vi "Vision Research Phantom Series PhCon PhSetCameraName.vi"(0 "CN in":u32=1, 2 "pCameraName":string, 5 "Error In (no error)":errorcluster) -> (14 "CN out":u32=1, 19 "Error Out":errorcluster)   [LabVIEW 2013, in "VRI.lvlib"]
doc: "PhCon.dll\n\nPhSetCameraName\nHRESULT PhSetCameraName(UINT CN, char *pCameraName);\n\nParameters Description\nCN (in) Camera number.\npCameraName (in) Camera name, maximum 15 char.\nReturn HRESULT (0=Ok)\nComments Let the user change the name of the camera.\n\nWritten by:\nBLOOMY CONTROLS, INC\nWINDSOR, CT 06095, USA\n860-298-9925\nwww.bloomy.com\nV1.0.0\nMay, 2004"
uses:
  VRI.lvlib
  Phantom DLLs/PhCon.dll
panel:
  # "For instructions on the use of this VI, press Ctrl+H to display the help window and move the mouse over the icon, controls, and indicators"
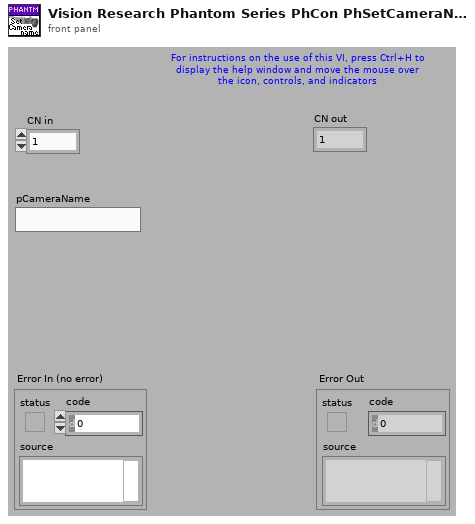
[diagram p1: front panel]
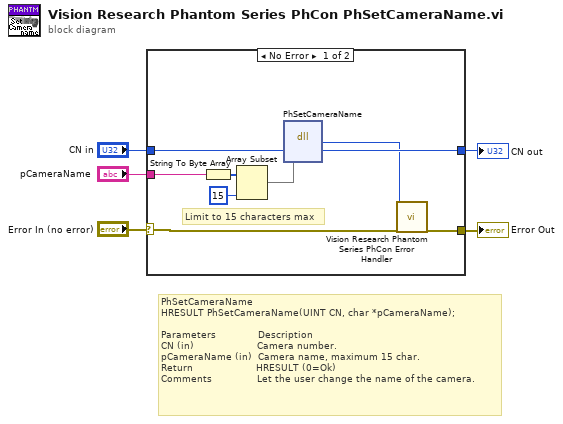
[diagram p0: block diagram]
diagram:
  # "PhSetCameraName\nHRESULT PhSetCameraName(UINT CN, char *pCameraName);\n\nParameters              Description\nCN (in)                     Camera number.\npCameraName (in)  Camera name, maximum 15 char.\nReturn                     HRESULT (0=Ok)\nComments               Let the user change the name of the camera."
  n1 = case shown="No Error" "Error In (no error)" {
    selector: "Error In (no error)" -> [w14 w16]
    tunnel: [w13 w16] -> w4
    tunnel: "CN in" -> [w12 w15]
    tunnel: "pCameraName" -> [w11 _]
    tunnel: [w10 w15] -> w1
    frame No Error {
      # "Limit to 15 characters max"
      n2 = String To Byte Array(string=w11) -> (unsigned byte array=w6:u8[])
      n3 = Array Subset(array=w6, length=15) -> (w8:u8[])  [unwired: 1 in]
      n4 = dll-call lib="C:/Projects/SDK/32-bit/Vision Research Phantom Series Labview Driver/Phantom DLLs/PhCon.dll" fn="PhSetCameraName"("CN"=w12, "pCameraName"=w8) -> ("HRESULT"=w9:i32, "CN"=w10:u32)  [unwired: 3 in, 3 out]
      n5 = call "Vision Research Phantom Series PhCon Error Handler.vi"("ErrNo"=w9, "Error In (no error)"=w14) -> ("Error Out"=w13:errorcluster)  [unwired: 17 out]
    }
    frame Error {
    }
  }
  "Error Out" <- w4
  "CN out" <- w1
